vi "LoopselFF_1_or_2cam_eventdriven.VI"() -> ()   [LabVIEW 2015]
uses:
  board.vis/Globals.vi
panel:
  in  "continuous":bool
  out "curr.block":dbl=3.0
  out "Measure ON":bool
  in  "cam select\n1: cam 1\n2: cam 2\n3: both cams":u8=3
  in  "no.of blocks (nob)\npress enter":u32=3
  in  "NOB":u32(slide)=1 max=10 scale=0.9..3.0
  out "Signalverlaufgraph 2":u16[](graph)=[0, 0, 543, 543, 0, 1, 0, 0, 2, 2, 3, 3, 4, 4, 5, 5, 6, 6, 7, 7, 8, 8, 9, 9, 10, 10, 11, 11, 12, 12, 13, 13, 14, 14, 15, 15, 16, 16, 17, 17, 18, 18, 19, 19, 20, 20, 21, 21, 22, 22, 23, 23, 24, 24, 25, 25, 26, 26, 27, 27, 28, 28, 29, 29, 30, 30, 31, 31, 32, 32, 33, 33, 34, 34, 35, 35, 36, 36, 37, 37, 38, 38, 39, 39, 40, 40, 41, 41, 42, 42, 43, 43, 44, 44, 45, 45, 46, 46, 47, 47, 48, 48, 49, 49, 50, 50, 51, 51, 52, 52, 53, 53, 54, 54, 55, 55, 56, 56, 57, 57, 58, 58, 59, 59, 60, 60, 61, 61, 62, 62, 63, 63, 64, 64, 65, 65, 66, 66, 67, 67, 68, 68, 69, 69, 70, 70, 71, 71, 72, 72, 73, 73, 74, 74, 75, 75, 76, 76, 77, 77, 78, 78, 79, 79, 80, 80, 81, 81, 82, 82, 83, 83, 84, 84, 85, 85, 86, 86, 87, 87, 88, 88, 89, 89, 90, 90, 91, 91, 92, 92, 93, 93, 94, 94, 95, 95, 96, 96, 97, 97, 98, 98, 99, 99, 100, 100, 101, 101, 102, 102, 103, 103, 104, 104, 105, 105, 106, 106, 107, 107, 108, 108, 109, 109, 110, 110, 111, 111, 112, 112, 113, 113, 114, 114, 115, 115, 116, 116, 117, 117, 118, 118, 119, 119, 120, 120, 121, 121, 122, 122, 123, 123, 124, 124, 125, 125, 126, 126, 127, 127, 128, 128, 129, 129, 130, 130, 131, 131, 132, 132, 133, 133, 134, 134, 135, 135, 136, 136, 137, 137, 138, 138, 139, 139, 140, 140, 141, 141, 142, 142, 143, 143, 144, 144, 145, 145, 146, 146, 147, 147, 148, 148, 149, 149, 150, 150, 151, 151, 152, 152, 153, 153, 154, 154, 155, 155, 156, 156, 157, 157, 158, 158, 159, 159, 160, 160, 161, 161, 162, 162, 163, 163, 164, 164, 165, 165, 166, 166, 167, 167, 168, 168, 169, 169, 170, 170, 171, 171, 172, 172, 173, 173, 174, 174, 175, 175, 176, 176, 177, 177, 178, 178, 179, 179, 180, 180, 181, 181, 182, 182, 183, 183, 184, 184, 185, 185, 186, 186, 187, 187, 188, 188, 189, 189, 190, 190, 191, 191, 192, 192, 193, 193, 194, 194, 195, 195, 196, 196, 197, 197, 198, 198, 199, 199, 200, 200, 201, 201, 202, 202, 203, 203, 204, 204, 205, 205, 206, 206, 207, 207, 208, 208, 209, 209, 210, 210, 211, 211, 212, 212, 213, 213, 214, 214, 215, 215, 216, 216, 217, 217, 218, 218, 219, 219, 220, 220, 221, 221, 222, 222, 223, 223, 224, 224, 225, 225, 226, 226, 227, 227, 228, 228, 229, 229, 230, 230, 231, 231, 232, 232, 233, 233, 234, 234, 235, 235, 236, 236, 237, 237, 238, 238, 239, 239, 240, 240, 241, 241, 242, 242, 243, 243, 244, 244, 245, 245, 246, 246, 247, 247, 248, 248, 249, 249, 250, 250, 251, 251, 252, 252, 253, 253, 254, 254, 255, 255, 256, 256, 257, 257, 258, 258, 259, 259, 260, 260, 261, 261, 262, 262, 263, 263, 264, 264, 265, 265, 266, 266, 267, 267, 268, 268, 269, 269, 270, 270, 271, 271, 272, 272, 273, 273, 274, 274, 275, 275, 276, 276, 277, 277, 278, 278, 279, 279, 280, 280, 281, 281, 282, 282, 283, 283, 284, 284, 285, 285, 286, 286, 287, 287, 288, 288, 289, 289, 290, 290, 291, 291, 292, 292, 293, 293, 294, 294, 295, 295, 296, 296, 297, 297, 298, 298, 299, 299, 300, 300, 301, 301, 302, 302, 303, 303, 304, 304, 305, 305, 306, 306, 307, 307, 308, 308, 309, 309, 310, 310, 311, 311, 312, 312, 313, 313, 314, 314, 315, 315, 316, 316, 317, 317, 318, 318, 319, 319, 320, 320, 321, 321, 322, 322, 323, 323, 324, 324, 325, 325, 326, 326, 327, 327, 328, 328, 329, 329, 330, 330, 331, 331, 332, 332, 333, 333, 334, 334, 335, 335, 336, 336, 337, 337, 338, 338, 339, 339, 340, 340, 341, 341, 342, 342, 343, 343, 344, 344, 345, 345, 346, 346, 347, 347, 348, 348, 349, 349, 350, 350, 351, 351, 352, 352, 353, 353, 354, 354, 355, 355, 356, 356, 357, 357, 358, 358, 359, 359, 360, 360, 361, 361, 362, 362, 363, 363, 364, 364, 365, 365, 366, 366, 367, 367, 368, 368, 369, 369, 370, 370, 371, 371, 372, 372, 373, 373, 374, 374, 375, 375, 376, 376, 377, 377, 378, 378, 379, 379, 380, 380, 381, 381, 382, 382, 383, 383, 384, 384, 385, 385, 386, 386, 387, 387, 388, 388, 389, 389, 390, 390, 391, 391, 392, 392, 393, 393, 394, 394, 395, 395, 396, 396, 397, 397, 398, 398, 399, 399, 400, 400, 401, 401, 402, 402, 403, 403, 404, 404, 405, 405, 406, 406, 407, 407, 408, 408, 409, 409, 410, 410, 411, 411, 412, 412, 413, 413, 414, 414, 415, 415, 416, 416, 417, 417, 418, 418, 419, 419, 420, 420, 421, 421, 422, 422, 423, 423, 424, 424, 425, 425, 426, 426, 427, 427, 428, 428, 429, 429, 430, 430, 431, 431, 432, 432, 433, 433, 434, 434, 435, 435, 436, 436, 437, 437, 438, 438, 439, 439, 440, 440, 441, 441, 442, 442, 443, 443, 444, 444, 445, 445, 446, 446, 447, 447, 448, 448, 449, 449, 450, 450, 451, 451, 452, 452, 453, 453, 454, 454, 455, 455, 456, 456, 457, 457, 458, 458, 459, 459, 460, 460, 461, 461, 462, 462, 463, 463, 464, 464, 465, 465, 466, 466, 467, 467, 468, 468, 469, 469, 470, 470, 471, 471, 472, 472, 473, 473, 474, 474, 475, 475, 476, 476, 477, 477, 478, 478, 479, 479, 480, 480, 481, 481, 482, 482, 483, 483, 484, 484, 485, 485, 486, 486, 487, 487, 488, 488, 489, 489, 490, 490, 491, 491, 492, 492, 493, 493, 494, 494, 495, 495, 496, 496, 497, 497, 498, 498, 499, 499, 500, 500, 501, 501, 502, 502, 503, 503, 504, 504, 505, 505, 506, 506, 507, 507, 508, 508, 509, 509, 510, 510, 511, 511, 512, 512, 513, 513, 514, 514, 515, 515, 516, 516, 517, 517, 518, 518, 519, 519, 520, 520, 521, 521, 522, 522, 523, 523, 524, 524, 525, 525, 526, 526, 527, 527, 528, 528, 529, 529, 530, 530, 531, 531, 532, 532, 533, 533, 534, 534, 535, 535, 536, 536, 537, 537, 538, 538, 539, 539, 540, 540, 541, 541]
  out "Signalverlaufgraph":u16[](graph)=[495, 495, 495, 495, 0, 1, 0, 31277, 13738, 13738, 16383, 16383, 16383, 16383, 16383, 16383, 16383, 16383, 16383, 16383, 16383, 16383, 16383, 16383, 16383, 16383, 16383, 16383, 16383, 16383, 16383, 16383, 16383, 16383, 16383, 16383, 16383, 16383, 16383, 16383, 16383, 16383, 16383, 16383, 16383, 16383, 16383, 16383, 16383, 16383, 16383, 16383, 16383, 16383, 16383, 16383, 16383, 16383, 16383, 16383, 16383, 16383, 16383, 16383, 16383, 16383, 16383, 16383, 16383, 16383, 16383, 16383, 16383, 16383, 16383, 16383, 16383, 16383, 16383, 16383, 16383, 16383, 16383, 16383, 16383, 16383, 16383, 16383, 16383, 16383, 16383, 16383, 16383, 16383, 16383, 16383, 16383, 16383, 16383, 16383, 16383, 16383, 16383, 16383, 16383, 16383, 16383, 16383, 16383, 16383, 16383, 16383, 16383, 16383, 16383, 16383, 16383, 16383, 16383, 16383, 16383, 16383, 16383, 16383, 16383, 16383, 16383, 16383, 16383, 16383, 16383, 16383, 16383, 16383, 16383, 16383, 16383, 16383, 15796, 16075, 15321, 16041, 15486, 16006, 16318, 16383, 16340, 16383, 16383, 16316, 16383, 16383, 16383, 16383, 16383, 16383, 16102, 15593, 16383, 16383, 16383, 16383, 16383, 16383, 16383, 16084, 16383, 16383, 15734, 16383, 16383, 16220, 15418, 15671, 16383, 16383, 16383, 16383, 16241, 16009, 15645, 16355, 15733, 16270, 16383, 16383, 15624, 16383, 16301, 16383, 16383, 16383, 16383, 16095, 16383, 15802, 16383, 15963, 16383, 16383, 16383, 16383, 16383, 16383, 16383, 16383, 16238, 15993, 16383, 15744, 16383, 15944, 16383, 16312, 16171, 16383, 15475, 16383, 16383, 15752, 16170, 16383, 16383, 16383, 15583, 15985, 16306, 16383, 15405, 16383, 16383, 16383, 16383, 15559, 16360, 15996, 15926, 16383, 16383, 16383, 15594, 16196, 16383, 16313, 16336, 16383, 16193, 15787, 16230, 16383, 16383, 16383, 16383, 16383, 16383, 16053, 15882, 15752, 16294, 15784, 15709, 16383, 16383, 16383, 14894, 14894, 16383, 16383, 16383, 16383, 16383, 16383, 16383, 16383, 16383, 16383, 16383, 16383, 16383, 16383, 16383, 16383, 16383, 16383, 16383, 16383, 16383, 16383, 16383, 16383, 16383, 16383, 16383, 16383, 16383, 16383, 16383, 16383, 16383, 16383, 16383, 16383, 16383, 16383, 16383, 16383, 16383, 16383, 16383, 16383, 16383, 16383, 16383, 16383, 16383, 16383, 16383, 16383, 16383, 16383, 16383, 16383, 16383, 16383, 16383, 16383, 16383, 16383, 16383, 16383, 16383, 16383, 16383, 16383, 16383, 16383, 16383, 16383, 16383, 16383, 16383, 16383, 16383, 16383, 16383, 16383, 16383, 16383, 16383, 16383, 16383, 16383, 16383, 16383, 16383, 16383, 16383, 16383, 16383, 16383, 16383, 16383, 16383, 16383, 16383, 16383, 16383, 16383, 16383, 16383, 16383, 16383, 16383, 16383, 16383, 16383, 16383, 16383, 16383, 16383, 16383, 16383, 16383, 16383, 16383, 16383, 16383, 16383, 16383, 16383, 16383, 16383, 16383, 16383, 16383, 16383, 16383, 16383, 16383, 16383, 16383, 16383, 16383, 16383, 16383, 16383, 16383, 16383, 16383, 16383, 16383, 16383, 16383, 16383, 16383, 16383, 16383, 16383, 16383, 16383, 16383, 16383, 16383, 16383, 16383, 16383, 16383, 16383, 16383, 16383, 16383, 16383, 16383, 16383, 16383, 16383, 16383, 16383, 16383, 16383, 16383, 16383, 16383, 16383, 16383, 16383, 16383, 16383, 16383, 16383, 16383, 16383, 16383, 16383, 16383, 16383, 16383, 16383, 16383, 16383, 16383, 16383, 16383, 16383, 16383, 16383, 16383, 16383, 16383, 16383, 16383, 16383, 16383, 16383, 16383, 16383, 16383, 16383, 16383, 16383, 16383, 16383, 16383, 16383, 16383, 16383, 16383, 16383, 16383, 16383, 16383, 16383, 16383, 16383, 16383, 16383, 16383, 16383, 16383, 16383, 16383, 16383, 16383, 16383, 16383, 16383, 16383, 16383, 16383, 16383, 16383, 16383, 16383, 16383, 16383, 16383, 16383, 16383, 16383, 16383, 16383, 16383, 16383, 16383, 16383, 16383, 16383, 16383, 16383, 16383, 16383, 16383, 16383, 16383, 16383, 16383, 16383, 16383, 16383, 16383, 16383, 16383, 16383, 16383, 16383, 16383, 16383, 16383, 16383, 16383, 16383, 16383, 16383, 16383, 16383, 16383, 16383, 16383, 16383, 16383, 16383, 16383, 16383, 16383, 16383, 16383, 16383, 16383, 16383, 16383, 16383, 16383, 16383, 16383, 16383, 16383, 16383, 16383, 16383, 16383, 16383, 16383, 16383, 16383, 16383, 16383, 16383, 16383, 16383, 16383, 16383, 16383, 16383, 16383, 16383, 16383, 16383, 16383, 16383, 16383, 16383, 16383, 16383, 16383, 16383, 16383, 16383, 16383, 16383, 16383, 16383, 16383, 16383, 16383, 16383, 16383, 16383, 16383, 16383, 16350, 16383, 16383, 16383, 16383, 16383, 16383, 16383, 16383, 16383, 16383, 16383, 16383, 16383, 16383, 16383, 16383, 16383, 16383, 16383, 16383, 16383, 16383, 16383, 16383, 16383, 16383, 16383, 16383, 16383, 16383, 16383, 16383, 16383, 16383, 16383, 16383, 16383, 16383, 16383, 16383, 16383, 16383, 16383, 16383, 16383, 16383, 16383, 16383, 16383, 16383, 16383, 16383, 16383, 16383, 16383, 16383, 16383, 16383, 16383, 16383, 16383, 16383, 16383, 16383, 16383, 16383, 16383, 16383, 16383, 16383, 16383, 16383, 16383, 16383, 16383, 16383, 16383, 16383, 16383, 16383, 16383, 16383, 16383, 16383, 16383, 16383, 16383, 16383, 16383, 16383, 16383, 16383, 16383, 16383, 16383, 16383, 16383, 16383, 16383, 16383, 16383, 16383, 16383, 16383, 16383, 16383, 16383, 16383, 16383, 16383, 16383, 16383, 16383, 16383, 16383, 16383, 16383, 16383, 16383, 16383, 16383, 16383, 16383, 16383, 16383, 16383, 16383, 16383, 16383, 16383, 16383, 16383, 16383, 16383, 16383, 16383, 16383, 16383, 16383, 16383, 16383, 16383, 16383, 16383, 16383, 16383, 16383, 16383, 16383, 16383, 16383, 16383, 16383, 16383, 16383, 16383, 16383, 16383, 16383, 16383, 16383, 16383, 16383, 16383, 16383, 16383, 16383, 16383, 16383, 16383, 16383, 16383, 16383, 16383, 16383, 16383, 16383, 16383, 16383, 16383, 16383, 16383, 16383, 16383, 16383, 16383, 16383, 16383, 16383, 16383, 16383, 16383, 16383, 16383, 16383, 16383, 16383, 16383, 16383, 16383, 16383, 16383, 16383, 16383, 16383, 16383, 16383, 16383, 16383, 16383, 16383, 16383, 16383, 16383, 16383, 16383, 16383, 16383, 16383, 16383, 16383, 16383, 16383, 16383, 16383, 16383, 16383, 16383, 16383, 16383, 16383, 16383, 16383, 16383, 16383, 16383, 16383, 16383, 16383, 16383, 16383, 16383, 16383, 16383, 16383, 16383, 16383, 16383, 16383, 16383, 16383, 16383, 16383, 16383, 16383, 16383, 16383, 16383, 16383, 16383, 16383, 16383, 16383, 16383, 16383, 16383, 16383, 16383, 16383, 16383, 16383, 16383, 16383, 16383, 16383, 16383, 16383, 16383, 16383, 16383, 16383, 16383, 16383, 16383, 16383, 16383, 13860, 13706, 14400, 14304, 14278, 14004, 14740, 14553, 13481, 13849, 13784, 14345, 14100, 13779, 14314, 14807, 14307, 13645, 14393, 14166, 13628, 14337, 13759, 13977, 14398, 14376, 13684, 14007, 14425, 14066, 13742, 14090, 14143, 14024, 14090, 14138, 13605, 13891, 13869, 13788, 13745, 13467, 13965, 14287, 14761, 14331, 13471, 14093, 14050, 14126, 13328, 14322, 14177, 13720, 13814, 13688, 13981, 13346, 13592, 13719, 14301, 14074, 14207, 13475, 14459, 13662, 14175, 13825, 13436, 14637, 13677, 13355, 14307, 13851, 14150, 14546, 14442, 13026, 13632, 13671, 13576, 14180, 14481, 13962, 13817, 14386, 14545, 13279, 14306, 14341, 13356, 13424, 13339, 14065, 13206, 13960, 13932, 14250, 14157, 14220, 14525, 13791, 13353, 13885, 14583, 13633, 13641, 14329, 13666, 13805, 14025, 14106, 13698, 13817, 13333, 14191, 14360, 14462, 14496, 14208, 14114, 13989, 14448, 14343, 14157, 1247, 978, 978, 589, 531, 510, 497, 497, 497, 497, 497, 497, 497, 497, 497, 497, 497, 497, 497, 497, 497, 497, 497, 497, 497, 497, 497, 497, 497, 497, 497, 497, 497, 497, 497, 497, 497, 497, 497, 497, 497, 497, 497, 497, 497, 497, 497, 497, 497, 497, 497, 497, 497, 497, 497, 497, 497]
  out "cams recognised":u8=1
  in  "alloc mem":bool
  out "FREE \nRAM MB":u64=13278
  out "BUILT-IN\nRAM MB":u64=16272
  out "SEC":dbl=3.6
  out "MB RAM":u64=374
  in  "pos slope":u8=1
  in  "both slopes":u8
  in  "DAT in 10ns":u32
  in  "extTrig  0/1\n0 : internal\n1:  \"I\" input (laser)":u8
  in  "stop all":bool
  in  "start":bool
  in  "NOS":u32(slide)=31278 max=3000 scale=1.0..6000.0
  in  "no.of samples (nos)":u32=6000
  in  "exposuretime[ms]":dbl=0.02 format="%.3f"
  # "Start with run"
  # "Abort with ESC"
  # "press Esc to stop measurement"
  # "exit here"
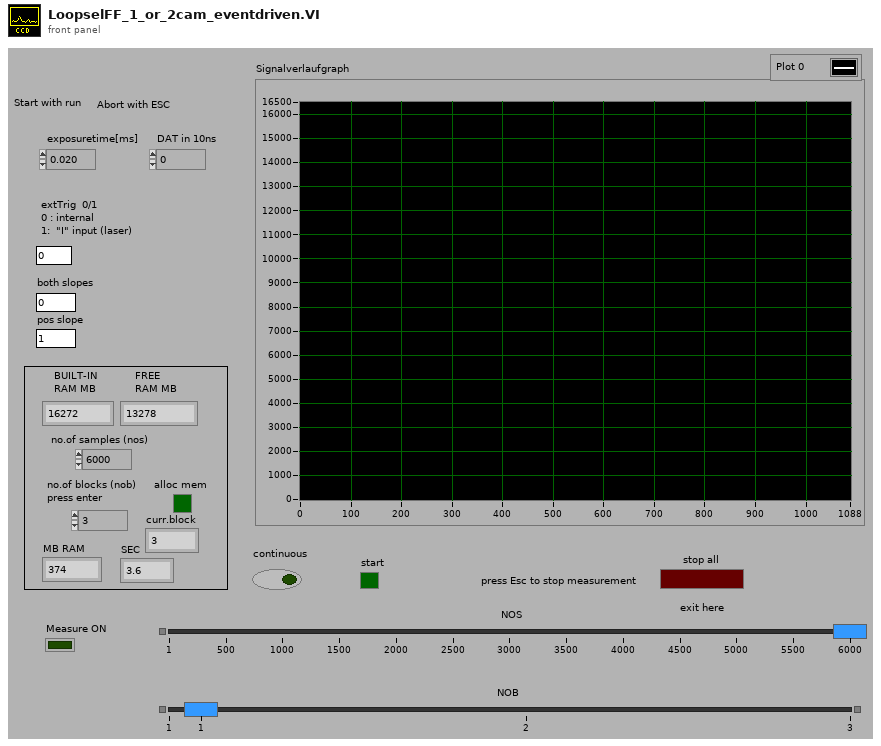
[diagram p1: front panel]
types:
  T1 = enum8{"Enabled", "Disabled", "Disabled and Grayed Out"}
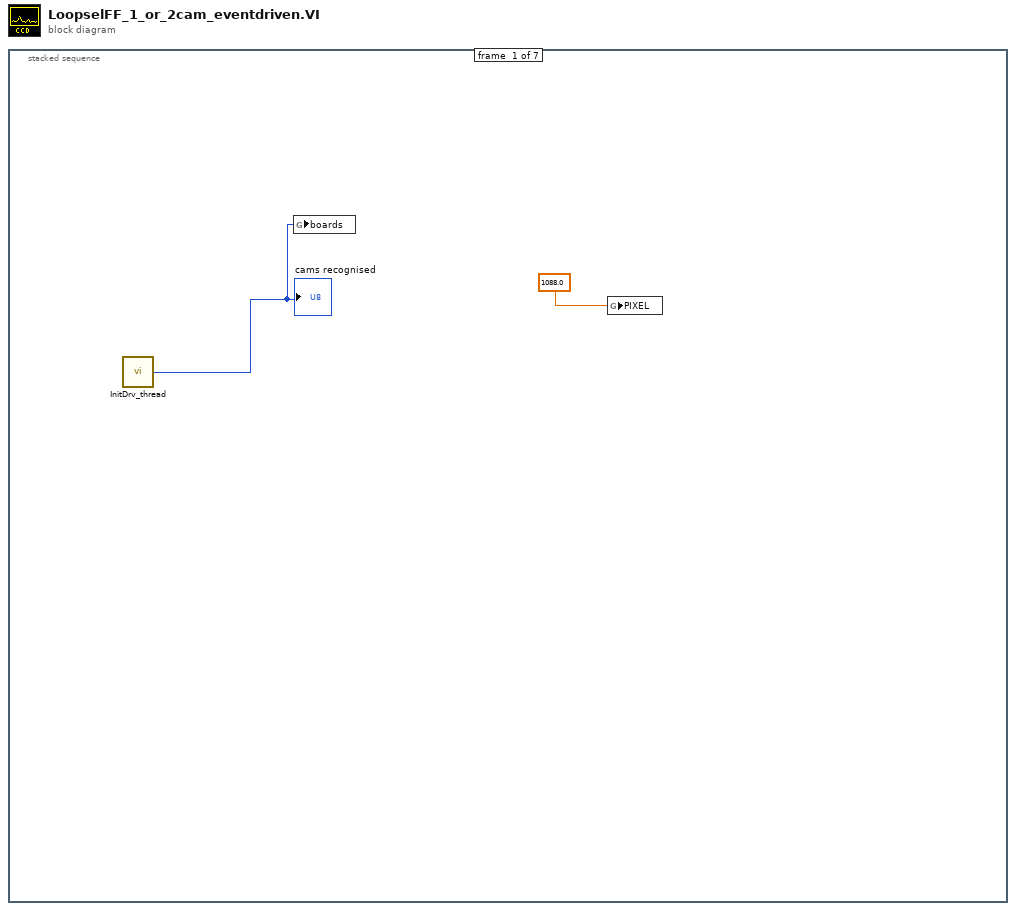
[diagram p0: block diagram]
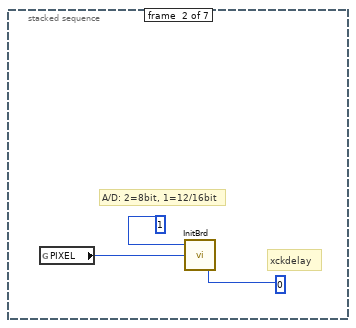
[diagram p2: hidden frame]
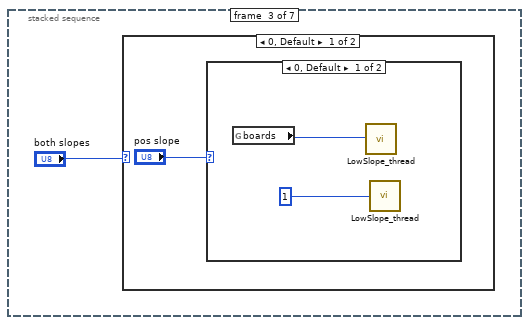
[diagram p3: hidden frame]
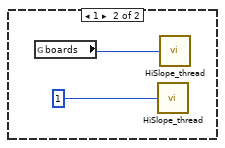
[diagram p4: hidden frame]
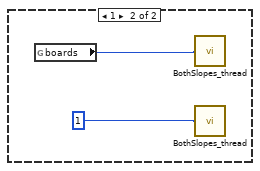
[diagram p5: hidden frame]
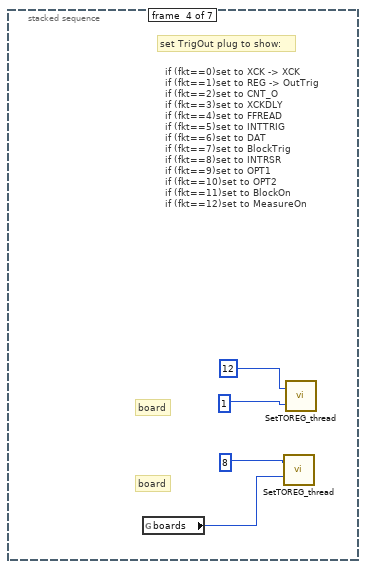
[diagram p6: hidden frame]
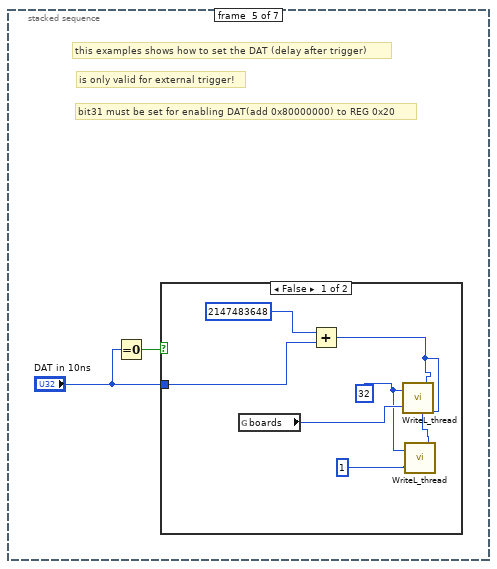
[diagram p7: hidden frame]
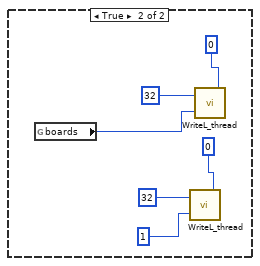
[diagram p8: hidden frame]
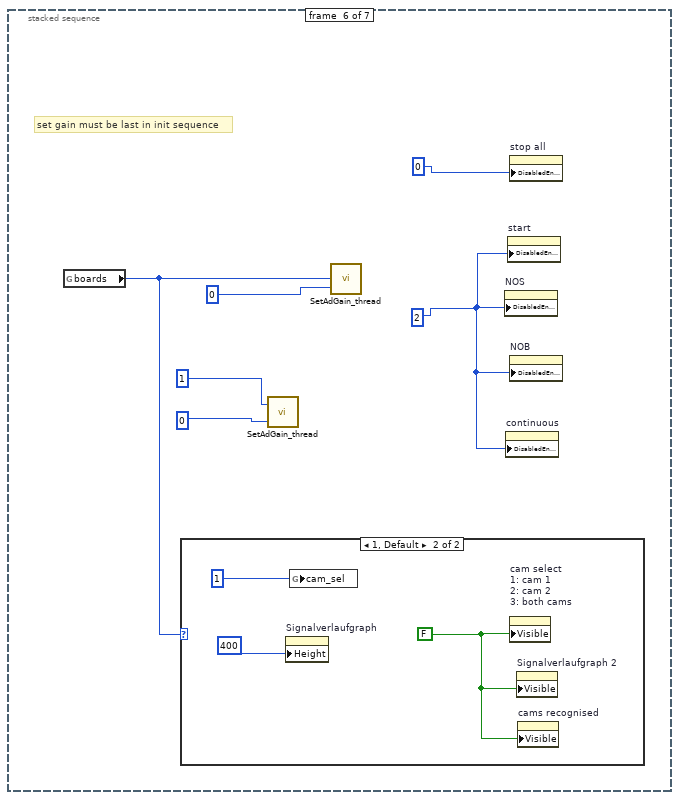
[diagram p9: hidden frame]
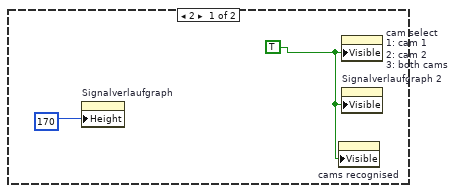
[diagram p10: hidden frame]
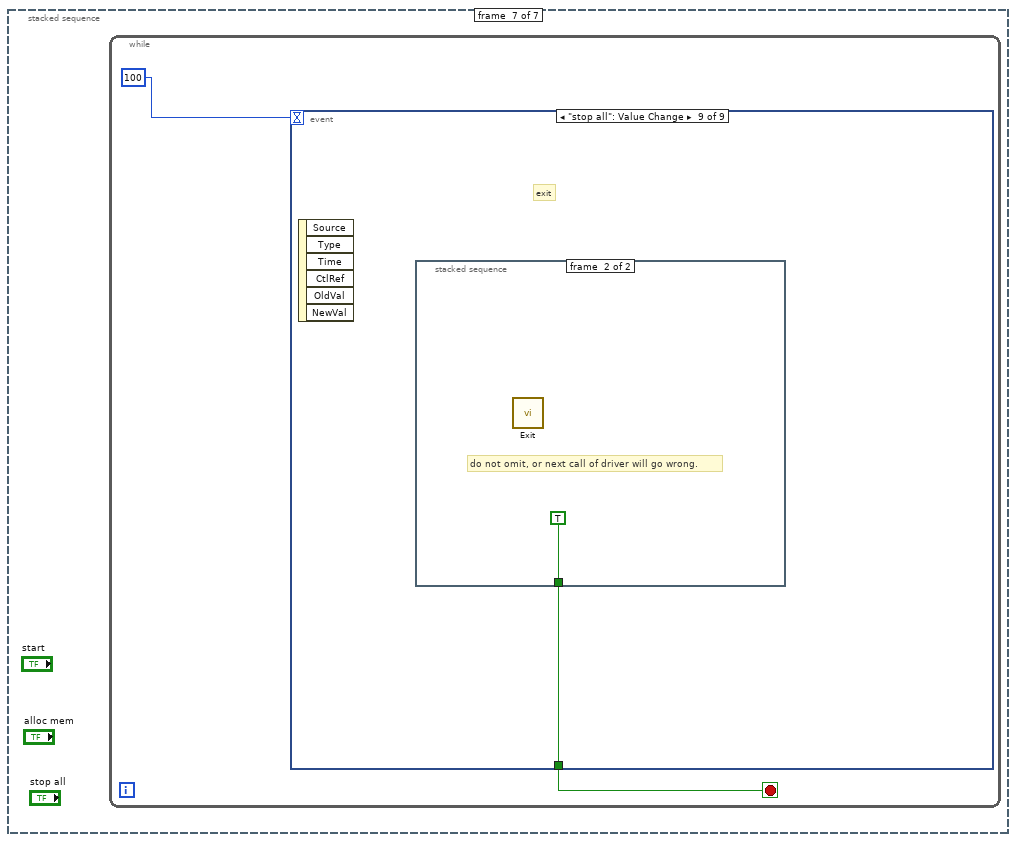
[diagram p11: hidden frame]
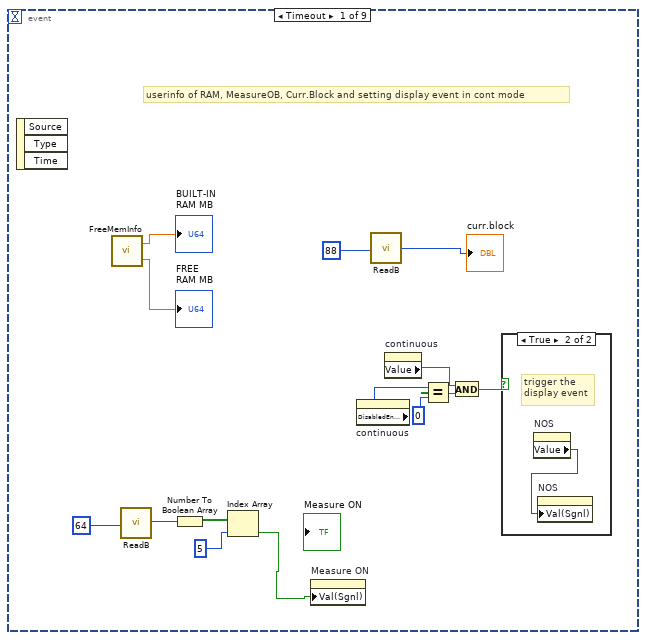
[diagram p12: hidden frame]
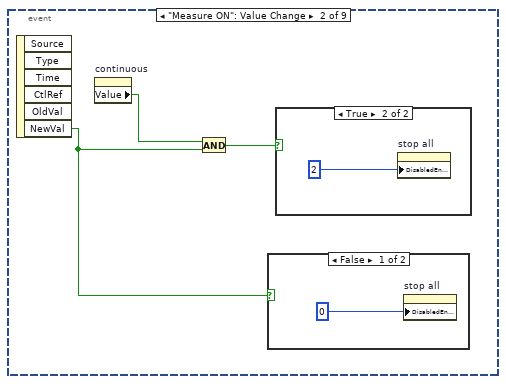
[diagram p14: hidden frame]
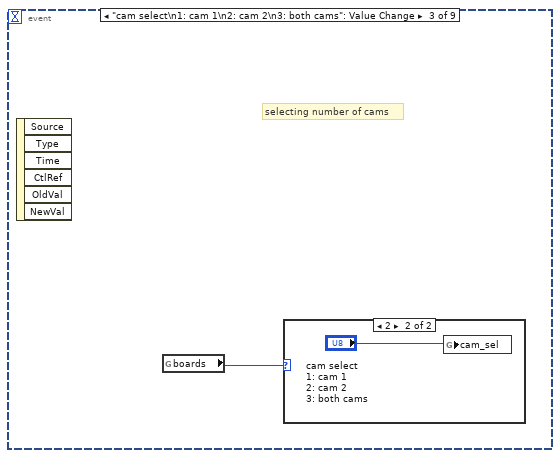
[diagram p17: hidden frame]
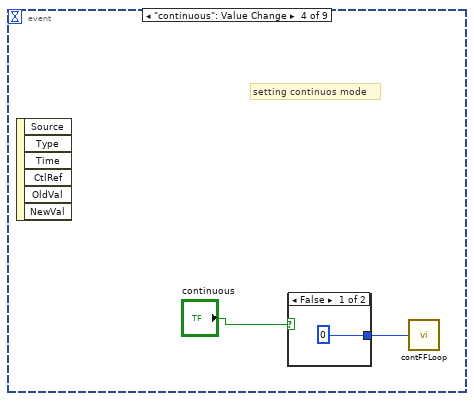
[diagram p19: hidden frame]
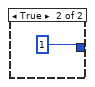
[diagram p20: hidden frame]
diagram:
  n1 = stacked-sequence {
    frame #0 {
      n2 = call "InitDrv_thread.vi"() -> ("Boards"=w1:u8)  [unwired: 1 in]
      "cams recognised" <- w1
      n3 = global write "Globals.vi" "boards"(w1) -> ()
      n4 = global write "Globals.vi" "PIXEL"(1088.0) -> ()
    }
    frame #1 {
      # "xckdelay"
      # "A/D: 2=8bit, 1=12/16bit"
      n5 = global read "Globals.vi" "PIXEL"() -> (w3:u32)
      n6 = call "InitBrd.vi"("xckdly"=u32 0, "pixel"=w3, "flag816"=u32 1) -> ()  [unwired: 3 in]
    }
    frame #2 {
      n7 = case shown="0, Default" "both slopes" {
        frame 0, Default {
          n8 = case shown="0, Default" "pos slope" {
            frame 0, Default {
              n9 = global read "Globals.vi" "boards"() -> (w8:u32)
              n10 = call "LowSlope_thread.vi"("board"=w8) -> ()  [unwired: 1 in]
              n11 = call "LowSlope_thread.vi"("board"=1) -> ()  [unwired: 1 in]
            }
            frame 1 {
              n12 = global read "Globals.vi" "boards"() -> (w11:u32)
              n13 = call "HiSlope_thread.vi"("board"=1) -> ()  [unwired: 1 in]
              n14 = call "HiSlope_thread.vi"("board"=w11) -> ()  [unwired: 1 in]
            }
          }
        }
        frame 1 {
          n15 = global read "Globals.vi" "boards"() -> (w13:u32)
          n16 = call "BothSlopes_thread.vi"("board"=w13) -> ()  [unwired: 1 in]
          n17 = call "BothSlopes_thread.vi"("board"=1) -> ()  [unwired: 1 in]
        }
      }
    }
    frame #3 {
      # "board"
      # "board"
      # "set TrigOut plug to show:"
      # "if (fkt==0)set to XCK -> XCK\nif (fkt==1)set to REG -> OutTrig\nif (fkt==2)set to CNT_O\nif (fkt==3)set to XCKDLY\nif (fkt==4)set to FFREAD\nif (fkt==5)set to INTTRIG\nif (fkt==6)set to DAT\nif (fkt==7)set to BlockTrig\nif (fkt==8)set to INTRSR\nif (fkt==9)set to OPT1\nif (fkt==10)set to OPT2\nif (fkt==11)set to BlockOn\nif (fkt==12)set to MeasureOn"
      n18 = global read "Globals.vi" "boards"() -> (w17:u32)
      n19 = call "SetTOREG_thread.vi"("board"=w17, "fkt"=u8 8) -> ()  [unwired: 1 in]
      n20 = call "SetTOREG_thread.vi"("board"=u8 1, "fkt"=u8 12) -> ()  [unwired: 1 in]
    }
    frame #4 {
      # "bit31 must be set for enabling DAT(add 0x80000000) to REG 0x20"
      # "is only valid for external trigger!"
      # "this examples shows how to set the DAT (delay after trigger)"
      n21 = Equal To 0?(x="DAT in 10ns") -> (x = 0?=w19:bool)
      n22 = case shown="False" w19 {
        tunnel: "DAT in 10ns" -> [w24 _]
        frame False {
          w21 = u32 32
          n23 = global read "Globals.vi" "boards"() -> (w23:u32)
          n24 = Add(x=u32 2147483648, y=w24) -> (x+y=w22:u32)
          n25 = call "WriteL_thread.vi"("val"=w22, "board"=w23, "offset"=w21) -> ()
          n26 = call "WriteL_thread.vi"("val"=w22, "board"=1, "offset"=w21) -> ()
        }
        frame True {
          n27 = global read "Globals.vi" "boards"() -> (w30:u32)
          n28 = call "WriteL_thread.vi"("val"=0, "board"=1, "offset"=u32 32) -> ()
          n29 = call "WriteL_thread.vi"("val"=0, "board"=w30, "offset"=u32 32) -> ()
        }
      }
    }
    frame #5 {
      w37 = 2
      # "set gain must be last in init sequence"
      n30 = global read "Globals.vi" "boards"() -> (w35:u32)
      n31 = case shown="1, Default" w35 {
        frame 2 {
          w39 = TRUE
          n32 = property on="Signalverlaufgraph" class="WFGraph (strict)"("Height"=u8 170) -> ()  [unwired: 2 in, 2 out]
          n33 = property on="cams recognised" class="DigNum (strict)"("Visible"=w39) -> ()  [unwired: 2 in, 2 out]
          n34 = property on="cam select\n1: cam 1\n2: cam 2\n3: both cams" class="DigNum (strict)"("Visible"=w39) -> ()  [unwired: 2 in, 2 out]
          n35 = property on="Signalverlaufgraph 2" class="WFGraph (strict)"("Visible"=w39) -> ()  [unwired: 2 in, 2 out]
        }
        frame 1, Default {
          w40 = FALSE
          n36 = property on="Signalverlaufgraph" class="WFGraph (strict)"("Height"=400) -> ()  [unwired: 2 in, 2 out]
          n37 = global write "Globals.vi" "cam_sel"(u8 1) -> ()
          n38 = property on="cam select\n1: cam 1\n2: cam 2\n3: both cams" class="DigNum (strict)"("Visible"=w40) -> ()  [unwired: 2 in, 2 out]
          n39 = property on="Signalverlaufgraph 2" class="WFGraph (strict)"("Visible"=w40) -> ()  [unwired: 2 in, 2 out]
          n40 = property on="cams recognised" class="DigNum (strict)"("Visible"=w40) -> ()  [unwired: 2 in, 2 out]
        }
      }
      n41 = call "SetAdGain_thread.vi"("gain"=u8 0, "board"=u32 1) -> ()  [unwired: 1 in]
      n42 = call "SetAdGain_thread.vi"("gain"=u8 0, "board"=w35) -> ()  [unwired: 1 in]
      n43 = property on="NOS" class="Slide (strict)"("DisabledEnum"=w37) -> ()  [unwired: 2 in, 2 out]
      n44 = property on="continuous" class="Bool (strict)"("DisabledEnum"=w37) -> ()  [unwired: 2 in, 2 out]
      n45 = property on="start" class="Bool (strict)"("DisabledEnum"=w37) -> ()  [unwired: 2 in, 2 out]
      n46 = property on="stop all" class="Bool (strict)"("DisabledEnum"=0) -> ()  [unwired: 2 in, 2 out]
      n47 = property on="NOB" class="Slide (strict)"("DisabledEnum"=w37) -> ()  [unwired: 2 in, 2 out]
    }
    frame #6 {
      n48 = while {
        stop <- w44 stop-if-true
        n49 = event shown="[8] \"stop all\": Value Change" {
          selector: _ -> [_ _ _ _ _ _ _ _ _]
          dyn-events: _ -> [_ _ _ _ _ _ _ _ _]
          timeout: 100 -> [_ _ _ _ _ _ _ _ _]
          tunnel: [_ _ _ _ _ _ _ _ w134] -> w44
          event Timeout {
            # "userinfo of RAM, MeasureOB, Curr.Block and setting display event in cont mode"
            n50 = event-data() -> ()  [unwired: 1 in, 3 out]
            n51 = call "FreeMemInfo.vi"() -> ("PhysicalSpace"=→"BUILT-IN\nRAM MB":dbl, "PhysicalFreeSpace"=→"FREE \nRAM MB":dbl)  [unwired: 1 in]
            n52 = call "ReadB.vi"("Offset"=64) -> ("Data"=w55:u8)
            n53 = Number To Boolean Array(number=w55) -> (Boolean array=w54:bool[])
            n54 = Index Array(array=w54, index=5) -> (element=w45:bool)
            n55 = property on="Measure ON" class="Bool (strict)"("Val(Sgnl)"=w45) -> ()  [unwired: 2 in, 2 out]
            n56 = property on="continuous" class="Bool (strict)"() -> ("DisabledEnum"=w47:T1)  [unwired: 2 in, 2 out]
            n57 = call "ReadB.vi"("Offset"=88) -> ("Data"=→"curr.block":u8)
            n58 = property on="continuous" class="Bool (strict)"() -> ("Value"=w50:bool)  [unwired: 2 in, 2 out]
            n59 = Equal?(x=w47, y=0) -> (x = y?=w48:bool)
            n60 = And(x=w50, y=w48) -> (x .and. y?=w49:bool)
            n61 = case shown="True" w49 {
              frame False {
              }
              frame True {
                # "trigger the \ndisplay event"
                n62 = property on="NOS" class="Slide (strict)"() -> ("Value"=w59:u32)  [unwired: 2 in, 2 out]
                n63 = property on="NOS" class="Slide (strict)"("Val(Sgnl)"=w59) -> ()  [unwired: 2 in, 2 out]
              }
            }
          }
          event "Measure ON": Value Change {
            n64 = event-data() -> ("NewVal"=w60:bool)  [unwired: 1 in, 5 out]
            n65 = property on="continuous" class="Bool (strict)"() -> ("Value"=w61:bool)  [unwired: 2 in, 2 out]
            n66 = And(x=w61, y=w60) -> (x .and. y?=w62:bool)
            n67 = case shown="False" w60 {
              frame False {
                n68 = property on="stop all" class="Bool (strict)"("DisabledEnum"=0) -> ()  [unwired: 2 in, 2 out]
              }
              frame True {
              }
            }
            n69 = case shown="True" w62 {
              frame False {
              }
              frame True {
                n70 = property on="stop all" class="Bool (strict)"("DisabledEnum"=2) -> ()  [unwired: 2 in, 2 out]
              }
            }
          }
          event "cam select\n1: cam 1\n2: cam 2\n3: both cams": Value Change {
            # "selecting number of cams"
            n71 = event-data() -> ()  [unwired: 1 in, 6 out]
            n72 = global read "Globals.vi" "boards"() -> (w65:u32)
            n73 = case shown="2" w65 {
              frame 0, Default {
              }
              frame 2 {
                n74 = global write "Globals.vi" "cam_sel"("cam select\n1: cam 1\n2: cam 2\n3: both cams") -> ()
              }
            }
          }
          event "continuous": Value Change {
            # "setting continuos mode"
            n75 = event-data() -> ()  [unwired: 1 in, 6 out]
            n76 = case shown="False" "continuous" {
              tunnel: [0 1] -> w67
              frame False {
              }
              frame True {
              }
            }
            n77 = call "contFFLoop.vi"("Numeric"=w67) -> ()  [unwired: 1 in]
          }
          event "alloc mem": Value Change {
            w75 = 0
            # "update params"
            # "Setup DMA"
            n78 = event-data() -> ()  [unwired: 1 in, 6 out]
            n79 = global read "Globals.vi" "nob"() -> (w73:u32)
            n80 = global read "Globals.vi" "boards"() -> (w76:u32)
            n81 = global read "Globals.vi" "nos"() -> (w72:u32)
            n82 = case shown="2" w76 {
              selector: w76 -> [_ w77]
              tunnel: w72 -> [_ w78]
              tunnel: w73 -> [_ w79]
              frame 1, Default {
              }
              frame 2 {
                # "Setup DMA"
                n83 = call "SetupDMA_thread.vi"("blocks"=w79, "nos"=w78, "Drv"=w77) -> ()  [unwired: 2 in]
              }
            }
            n84 = call "SetupDMA_thread.vi"("blocks"=w73, "nos"=w72, "Drv"=u32 1) -> ()  [unwired: 2 in]
            n85 = property on="continuous" class="Bool (strict)"("DisabledEnum"=w75) -> ()  [unwired: 2 in, 2 out]
            n86 = property on="NOB" class="Slide (strict)"("DisabledEnum"=w75) -> ()  [unwired: 2 in, 2 out]
            n87 = property on="NOS" class="Slide (strict)"("DisabledEnum"=w75) -> ()  [unwired: 2 in, 2 out]
            n88 = property on="exposuretime[ms]" class="DigNum (strict)"() -> ("Value"=w74:dbl)  [unwired: 2 in, 2 out]
            n89 = property on="start" class="Bool (strict)"("DisabledEnum"=w75) -> ()  [unwired: 2 in, 2 out]
            n90 = property on="exposuretime[ms]" class="DigNum (strict)"("Val(Sgnl)"=w74) -> ()  [unwired: 2 in, 2 out]
          }
          event "start": Mouse Down {
            # "start measurement"
            # "only 1st PCI board is used for ext. trig."
            # "ext. block trig\n0: internal: Space\n1: PCI \"I\"\n2: S1\n3: S2"
            # "block trigger 0/1\n0: internal -> next block is started immediately \n1: external -> each block has an own trigger"
            n91 = event-data() -> ()  [unwired: 1 in, 8 out]
            n92 = global read "Globals.vi" "exp time"() -> (w85:dbl)
            n93 = Multiply(x=1000.0, y=w85) -> (x*y=w87:dbl)
            n94 = global read "Globals.vi" "cam_sel"() -> (w80:u8)
            n95 = To Unsigned Long Integer(number=w87) -> (unsigned 32bit integer=w82:u32)
            n96 = call "ReadFFLoop_thread.vi"("blocktrigger"=u8 0, "btrig_ch"=u8 0, "ExtTrig"="extTrig  0/1\n0 : internal\n1:  \"I\" input (laser)", "cam_sel"=w80, "exptus"=w82) -> ()  [unwired: 1 in]
          }
          event "NOS", "NOB": Value Change {
            w97 = 1
            # "display"
            n97 = event-data() -> ()  [unwired: 1 in, 6 out]
            n98 = global read "Globals.vi" "boards"() -> (w100:u32)
            n99 = global read "Globals.vi" "nob"() -> (w89:u32)
            n100 = global read "Globals.vi" "nos"() -> (w96:u32)
            n101 = Greater?(x=w89, y="NOB") -> (0:w92:bool)
            n102 = Greater?(x=w96, y="NOS") -> (0:w95:bool)
            n103 = global read "Globals.vi" "PIXEL"() -> (w104:u32)
            n104 = case shown="True" w92 {
              tunnel: [1 w106] -> w91
              tunnel: "NOB" -> [_ w106]
              frame False {
              }
              frame True {
              }
            }
            n105 = case shown="False" w95 {
              tunnel: [1 w108] -> w94
              tunnel: "NOS" -> [_ w108]
              frame False {
              }
              frame True {
              }
            }
            n106 = Initialize Array(100, w104) -> (w103:i32[])
            n107 = Subtract(x=w94, y=w97) -> (x-y=w99:u32)
            n108 = Subtract(x=w91, y=w97) -> (x-y=w98:u32)
            n109 = case shown="2" w100 {
              selector: w100 -> [_ w111]
              tunnel: w99 -> [_ w112]
              tunnel: w98 -> [_ w109]
              frame 0, Default {
              }
              frame 2 {
                n110 = global read "Globals.vi" "PIXEL"() -> (w115:u32)
                n111 = Initialize Array(100, w115) -> (w114:i32[])
                n112 = call "ReturnFrame.vi"("Data Values In"=w114, "curr_nob"=w109, "curr_nos"=w112, "Drv"=w111) -> ("Data Values Out"=→"Signalverlaufgraph 2":u16[])  [unwired: 1 in]
              }
            }
            n113 = call "ReturnFrame.vi"("Data Values In"=w103, "curr_nob"=w98, "curr_nos"=w99, "Drv"=1) -> ("Data Values Out"=→"Signalverlaufgraph":u16[])  [unwired: 1 in]
          }
          event "no.of samples (nos)", "no.of blocks (nob)\npress enter", "exposuretime[ms]": Value Change {
            # "calculation of MB RAM an SEC and setting scale max"
            # "MB"
            # "ushort"
            n114 = event-data() -> ()  [unwired: 1 in, 6 out]
            n115 = global read "Globals.vi" "PIXEL"() -> (w133:u32)
            n116 = global read "Globals.vi" "boards"() -> (w132:u32)
            n117 = Multiply(x="no.of samples (nos)", y=w133) -> (x*y=w129:u32)
            n118 = Multiply(x=w129, y=2.0) -> (x*y=w130:dbl)
            n119 = global read "Globals.vi" "nos"() -> (w116:u32)
            n120 = global read "Globals.vi" "nob"() -> (w117:u32)
            n121 = Multiply(x=w130, y=w132) -> (x*y=w131:dbl)
            n122 = Divide(x=w131, y=1048576.0) -> (x/y=w121:dbl)
            n123 = property on="NOS" class="Slide (strict)"("Scale.Maximum"=w116) -> ()  [unwired: 2 in, 2 out]
            n124 = property on="NOB" class="Slide (strict)"("Scale.Maximum"=w117) -> ()  [unwired: 2 in, 2 out]
            n125 = Multiply(x=w121, y="no.of blocks (nob)\npress enter") -> (x*y=→"MB RAM":dbl)
            n126 = global write "Globals.vi" "nos"("no.of samples (nos)") -> ()
            n127 = Multiply(x="no.of samples (nos)", y="no.of blocks (nob)\npress enter") -> (x*y=w120:u32)
            n128 = global write "Globals.vi" "nob"("no.of blocks (nob)\npress enter") -> ()
            n129 = Multiply(x="exposuretime[ms]", y=w120) -> (x*y=w127:dbl)
            n130 = global write "Globals.vi" "exp time"("exposuretime[ms]") -> ()
            n131 = Divide(x=w127, y=1000) -> (x/y=→"SEC":dbl)
          }
          event "stop all": Value Change {
            # "exit"
            n132 = event-data() -> ()  [unwired: 1 in, 6 out]
            n133 = stacked-sequence {
              tunnel: [_ TRUE] -> w134
              frame #0 {
                n134 = call "FFStop.vi"() -> ()  [unwired: 1 in]
              }
              frame #1 {
                # "do not omit, or next call of driver will go wrong."
                n135 = call "Exit.vi"() -> ()  [unwired: 1 in]
              }
            }
          }
        }
      }
    }
  }
